vi "Set CRD Laser Params.vi"() -> ()   [LabVIEW 2017]
panel:
  out "(hi.lo)":u32
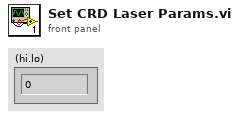
[diagram p1: front panel]
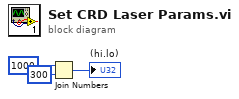
[diagram p0: block diagram]
diagram:
  n1 = Join Numbers(hi=u16 1000, lo=u16 300) -> ((hi.lo)=→"(hi.lo)":u32)
